vi "From Variant.vi"(8 "Error In":errorcluster, 10 "Variant":variant, 11 "Tree Data Type":refnum<class "Tree Data.lvclass">) -> (0 "Error Out":errorcluster, 3 "Tree Data Out":refnum<class "Tree Data.lvclass">)   [LabVIEW 2020, in "NI_VIAnCFGDataStructure.lvlib" / "Tree.lvclass"]
doc: "Converts the LV Variant data into Tree Data type. If your type is not one of the basic Tree Data types you can wire it to the Tree Data Type input to inform the converter which dynamically dispatched method to use for conversion.\n\n<b>WARNING</b> Do not use this method for conversion of clusters since they are complex types. Instead use the Cluster To Tree conversion method that builds a Tree from a cluster.\n\n<b>Supported basic types are:</b>\nBoolean, Boolean 1D Array, Boolean 2D Array\nInteger, Integer 1D Array, Integer 2D Array (I8, I16, I32, I64, U8, U16, U32, U64, Enum U8, Enum U16, Enum U32, Enum U64)\nFloat, Float 1D Array, Float 2D Array (Single, Double, Single with Unit, Double with Unit)\nString, String 1D Array, String 2D Array\nPath, Path 1D Array, Path 2D Array\n\nTo support more types you need to create your own conversion by overriding the dynamically dispatched To Variant and From Variant methods."
uses:
  <vilib>/addons/analyzer/VIAnCFGDataStructure/Tree Manager/Tree.lvclass
  <vilib>/addons/analyzer/VIAnCFGDataStructure/Tree Data/Tree Data.lvclass
  <vilib>/addons/analyzer/VIAnCFGDataStructure/Data Types/Int/Int.lvclass
  e:/builds/penguin/labview/branches/2020/dev/dist/vi.lib/addons/analyzer/VIAnCFGDataStructure/Tree Data/Tree Data.lvclass
  <vilib>/addons/analyzer/VIAnCFGDataStructure/Data Types/Float/Flt.lvclass
  <vilib>/addons/analyzer/VIAnCFGDataStructure/Data Types/Bool/Bool.lvclass
  <vilib>/addons/analyzer/VIAnCFGDataStructure/Data Types/String/String.lvclass
  <vilib>/addons/analyzer/VIAnCFGDataStructure/Data Types/Path/Path.lvclass
  <vilib>/addons/analyzer/VIAnCFGDataStructure/Data Types/Int Array/1D Int.lvclass
  <vilib>/addons/analyzer/VIAnCFGDataStructure/Data Types/Flt Array/1D Flt.lvclass
  <vilib>/addons/analyzer/VIAnCFGDataStructure/Data Types/Bool Array/1D Bool.lvclass
  <vilib>/addons/analyzer/VIAnCFGDataStructure/Data Types/String Array/1D String.lvclass
  <vilib>/addons/analyzer/VIAnCFGDataStructure/Data Types/Path Array/1D Path.lvclass
  <vilib>/addons/analyzer/VIAnCFGDataStructure/Data Types/2D Int/2D Int.lvclass
  <vilib>/addons/analyzer/VIAnCFGDataStructure/Data Types/2D Flt/2D Flt.lvclass
  <vilib>/addons/analyzer/VIAnCFGDataStructure/Data Types/2D Bool/2D Bool.lvclass
  <vilib>/addons/analyzer/VIAnCFGDataStructure/Data Types/2D String/2D String.lvclass
  <vilib>/addons/analyzer/VIAnCFGDataStructure/Data Types/2D Path/2D Path.lvclass
  <vilib>/Utility/error.llb/Error Cluster From Error Code.vi
  <vilib>/ErrorRing/Error Ring.xnode
  <vilib>/Utility/Data Type/NI_Data Type.lvlib
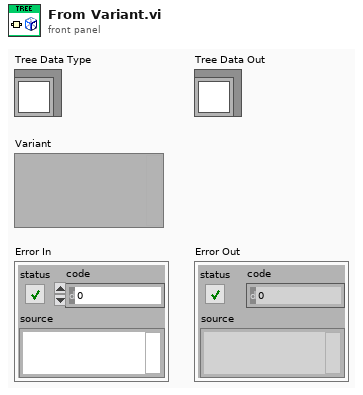
[diagram p1: front panel]
types:
  T1 = typedef "NI_Data Type.lvlib/Data Type.ctl" = enum8{"Invalid Type", "Void", "I8", "I16", "I32", "I64", "U8", "U16", "U32", "U64", "Single Float", "Double Float", "Extended Float", "Single Complex", "Double Complex", "Extended Complex", "Enum U8", "Enum U16", "Enum U32", "Enum U64", "Single Float With Unit", "Double Float With Unit", "Extended Float With Unit", "Single Complex with Unit", "Double Complex with Unit", "Extended Complex with Unit", "Boolean", "String", "Path", "Picture", "Tag", "Array", "Cluster", "Variant", "LV Variant", "Waveform", "Timestamp", "Digital Waveform", "Digital Data", "ExpressData", "Refnum", "External Data", "VI", "Poly VI", "LabVIEW Class Instance", "Fixed Point", "Set Collection", "Map Collection"}
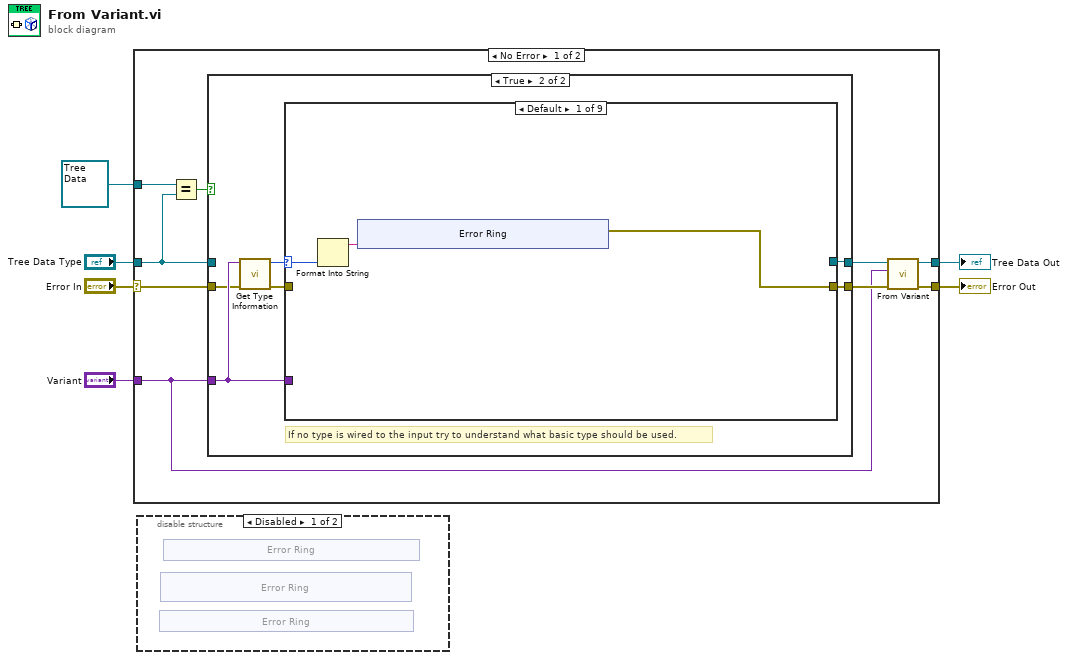
[diagram p0: block diagram]
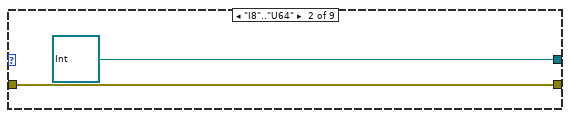
[diagram p3: hidden frame]
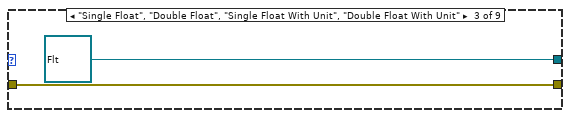
[diagram p4: hidden frame]
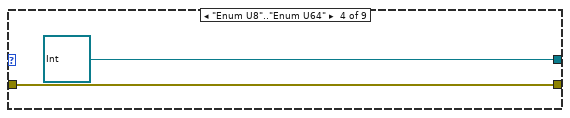
[diagram p5: hidden frame]
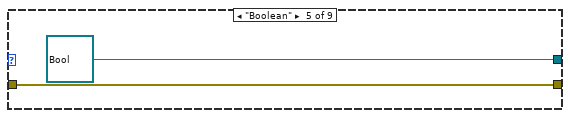
[diagram p6: hidden frame]
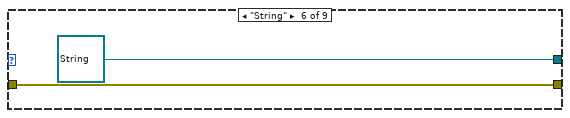
[diagram p7: hidden frame]
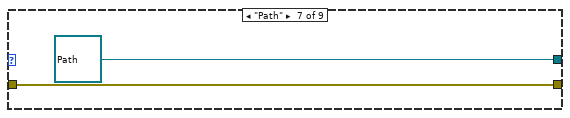
[diagram p8: hidden frame]
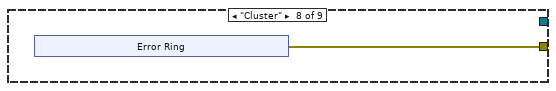
[diagram p9: hidden frame]
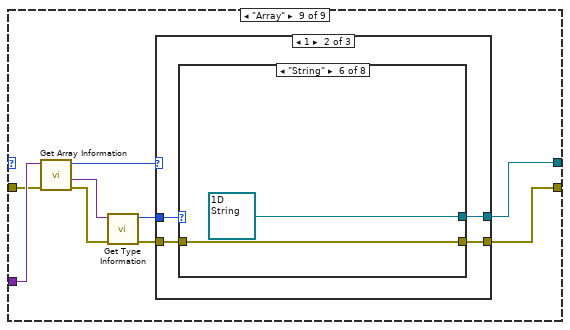
[diagram p10: hidden frame]
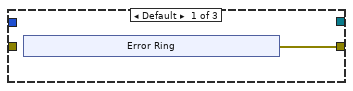
[diagram p11: hidden frame]
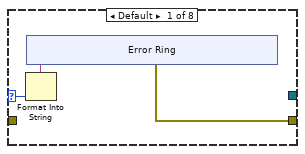
[diagram p12: hidden frame]
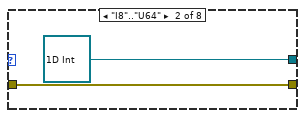
[diagram p13: hidden frame]
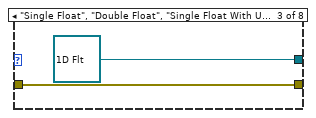
[diagram p14: hidden frame]
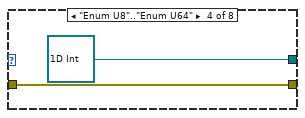
[diagram p15: hidden frame]
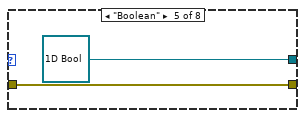
[diagram p16: hidden frame]
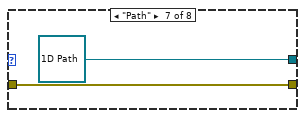
[diagram p17: hidden frame]
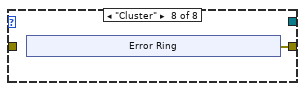
[diagram p18: hidden frame]
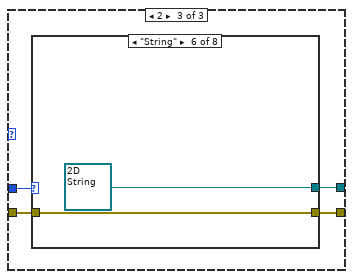
[diagram p19: hidden frame]
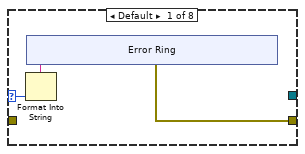
[diagram p20: hidden frame]
diagram:
  n1 = case shown="No Error" "Error In" {
    selector: "Error In" -> [w15 w131]
    tunnel: "Variant" -> [w7 _]
    tunnel: [w10 _] -> w5
    tunnel: [w9 w131] -> w4
    tunnel: "Tree Data Type" -> [w13 _]
    tunnel: refnum<class "Tree Data.lvclass"> refnum ("x") -> [w12 _]
    frame No Error {
      n2 = Equal?(x=w12, y=w13) -> (x = y?=w14:bool)
      n3 = case shown="True" w14 {
        tunnel: w7 -> [_ w23]
        tunnel: [w17 w19] -> w11
        tunnel: [w16 w18] -> w8
        tunnel: w15 -> [w16 w20]
        tunnel: w13 -> [w17 _]
        frame False {
          # "If a type is wired to the input use it as a definition on how to unflatten the variant."
        }
        frame True {
          # "If no type is wired to the input try to understand what basic type should be used."
          n4 = call <vilib>:"Get Type Information.vi"("error in (no error)"=w20, "variant"=w23) -> ("error out"=w22:errorcluster, "type"=w21:T1)  [unwired: 5 in, 3 out]
          n5 = case shown="Default" w21 {
            selector: w21 -> [w26 _ _ _ _ _ _ _ _]
            tunnel: w22 -> [_ w34 w36 w38 w40 w42 w44 _ w52]
            tunnel: w23 -> [_ _ _ _ _ _ _ _ w53]
            tunnel: [_ refnum<class "Int.lvclass"> refnum ("Int.lvclass") refnum<class "Flt.lvclass"> refnum ("Flt.lvclass") refnum<class "Int.lvclass"> refnum ("Int.lvclass") refnum<class "Bool.lvclass"> refnum ("TD Bool.lvclass") refnum<class "String.lvclass"> refnum ("TD String.lvclass") refnum<class "Path.lvclass"> refnum ("TD Path.lvclass") _ w55] -> w19
            tunnel: [w24 w34 w36 w38 w40 w42 w44 w46 w54] -> w18
            frame Default {
              n6 = Format Into String(w26) -> (resulting string=w25:string)  [unwired: 3 in, 1 out]
              n7 = xnode "Error Ring"("parameter 0"=w25) -> ("error out"=w24:errorcluster)
            }
            frame "I8".."U64" {
            }
            frame "Single Float", "Double Float", "Single Float With Unit", "Double Float With Unit" {
            }
            frame "Enum U8".."Enum U64" {
            }
            frame "Boolean" {
            }
            frame "String" {
            }
            frame "Path" {
            }
            frame "Cluster" {
              n8 = xnode "Error Ring"() -> ("error out"=w46:errorcluster)
            }
            frame "Array" {
              n9 = call <vilib>:"Get Array Information.vi"("error in (no error)"=w52, "variant"=w53) -> ("error out"=w58:errorcluster, "array element data type"=w56:variant, "number of dimensions"=w60:i32)  [unwired: 6 in, 1 out]
              n10 = call <vilib>:"Get Type Information.vi"("error in (no error)"=w58, "variant"=w56) -> ("error out"=w59:errorcluster, "type"=w57:T1)  [unwired: 5 in, 3 out]
              n11 = case shown="1" w60 {
                tunnel: w57 -> [_ w70 w102]
                tunnel: w59 -> [_ w67 w99]
                tunnel: [_ w68 w100] -> w55
                tunnel: [w61 w69 w101] -> w54
                frame Default {
                  n12 = xnode "Error Ring"() -> ("error out"=w61:errorcluster)
                }
                frame 1 {
                  n13 = case shown="\"String\"" w70 {
                    selector: w70 -> [w73 _ _ _ _ _ _ _]
                    tunnel: [_ refnum<class "1D Int.lvclass"> refnum ("Int Array.lvclass") refnum<class "1D Flt.lvclass"> refnum ("Flt Array.lvclass") refnum<class "1D Int.lvclass"> refnum ("TD Int A.lvclass") refnum<class "1D Bool.lvclass"> refnum ("TD Bool A.lvclass") refnum<class "1D String.lvclass"> refnum ("TD String A.lvclass") refnum<class "1D Path.lvclass"> refnum ("TD Path A.lvclass") _] -> w68
                    tunnel: [w71 w82 w84 w86 w88 w90 w92 w93] -> w69
                    tunnel: w67 -> [_ w82 w84 w86 w88 w90 w92 _]
                    frame Default {
                      n14 = Format Into String(w73) -> (resulting string=w72:string)  [unwired: 3 in, 1 out]
                      n15 = xnode "Error Ring"("parameter 0"=w72) -> ("error out"=w71:errorcluster)
                    }
                    frame "I8".."U64" {
                    }
                    frame "Single Float", "Double Float", "Single Float With Unit", "Double Float With Unit" {
                    }
                    frame "Enum U8".."Enum U64" {
                    }
                    frame "Boolean" {
                    }
                    frame "String" {
                    }
                    frame "Path" {
                    }
                    frame "Cluster" {
                      n16 = xnode "Error Ring"() -> ("error out"=w93:errorcluster)
                    }
                  }
                }
                frame 2 {
                  n17 = case shown="\"String\"" w102 {
                    selector: w102 -> [w105 _ _ _ _ _ _ _]
                    tunnel: [_ refnum<class "2D Int.lvclass"> refnum ("Tree API.lvlib:2D Int.lvclass") refnum<class "2D Flt.lvclass"> refnum ("Tree API.lvlib:2D Flt.lvclass") refnum<class "2D Int.lvclass"> refnum ("Tree API.lvlib:2D Int.lvclass") refnum<class "2D Bool.lvclass"> refnum ("Tree API.lvlib:2D Bool.lvclass") refnum<class "2D String.lvclass"> refnum ("Tree API.lvlib:2D String.lvclass") refnum<class "2D Path.lvclass"> refnum ("Tree API.lvlib:2D Path.lvclass") _] -> w100
                    tunnel: [w103 w114 w116 w118 w120 w122 w124 w125] -> w101
                    tunnel: w99 -> [_ w114 w116 w118 w120 w122 w124 _]
                    frame Default {
                      n18 = Format Into String(w105) -> (resulting string=w104:string)  [unwired: 3 in, 1 out]
                      n19 = xnode "Error Ring"("parameter 0"=w104) -> ("error out"=w103:errorcluster)
                    }
                    frame "I8".."U64" {
                    }
                    frame "Single Float", "Double Float", "Single Float With Unit", "Double Float With Unit" {
                    }
                    frame "Enum U8".."Enum U64" {
                    }
                    frame "Boolean" {
                    }
                    frame "String" {
                    }
                    frame "Path" {
                    }
                    frame "Cluster" {
                      n20 = xnode "Error Ring"() -> ("error out"=w125:errorcluster)
                    }
                  }
                }
              }
            }
          }
        }
      }
      n21 = call-dynamic "From Variant.vi"("Error In"=w8, "Variant"=w7, "Tree Data In"=w11) -> ("Error Out"=w9:errorcluster, "Tree Data Out"=w10:refnum<class "Tree Data.lvclass">)  [unwired: 7 in]
    }
    frame Error {
    }
  }
  "Error Out" <- w4
  "Tree Data Out" <- w5
  n22 = disable-structure shown="Disabled" {
    frame Disabled {
      n23 = xnode "Error Ring"() -> ()  [unwired: 1 out]
      n24 = xnode "Error Ring"() -> ()  [unwired: 1 in, 1 out]
      n25 = xnode "Error Ring"() -> ()  [unwired: 1 out]
    }
    frame Enabled {
    }
  }
